vi "Default Settings.vi"(8 "error in (no error)":errorcluster, 11 "8 Inch CAD Dispense in":refnum<class "8 Inch CAD Dispense.lvclass">) -> (0 "error out":errorcluster, 3 "8 Inch CAD Dispense out":refnum<class "8 Inch CAD Dispense.lvclass">)   [LabVIEW 2016, in "8 Inch CAD Dispense.lvclass"]
uses:
  8 Inch CAD Dispense.lvclass
  D:/LabVIEW/20220413/UCSB-Gantry/V5/Classes/Routine/Dispense/CAD Dispense/CAD Dispense.lvclass
  D:/LabVIEW/20220413/UCSB-Gantry/V5/Classes/Routine/Dispense/Dispense.lvclass
  CAD Dispense.lvclass/CAD Dispense.ctl
  Read Glue Speed.vi
  Read Move Speed.vi
  CAD Dispense.lvclass
  Dispense.lvclass
panel:
  # "This Routine does not Accept Settings"
  # "This Routine Does not Accept Settings"
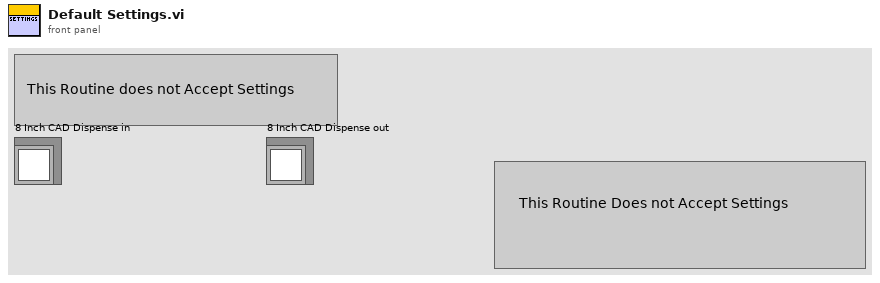
[diagram p1: front panel]
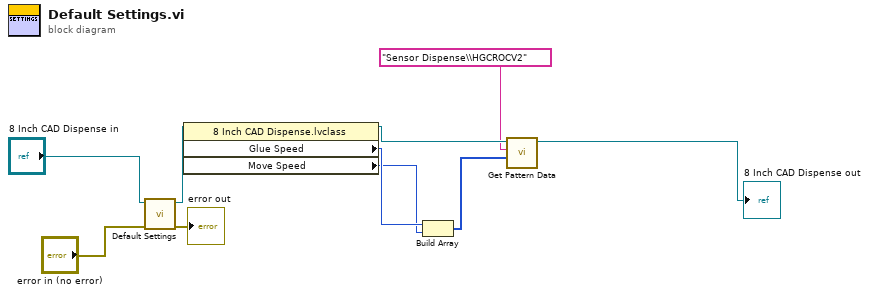
[diagram p0: block diagram]
diagram:
  n1 = call-parent "Default Settings.vi"("error in (no error)"="error in (no error)", "CAD Dispense in"="8 Inch CAD Dispense in") -> ("error out"=→"error out":errorcluster, "CAD Dispense out"=w7:refnum<class "8 Inch CAD Dispense.lvclass">)  [unwired: 8 in]
  n2 = property class="8 Inch CAD Dispense.lvclass"(reference=w7) -> (reference out=w3:refnum<class "8 Inch CAD Dispense.lvclass">, "Glue Speed"=w6:i32, "Move Speed"=w5:i32)  [unwired: 1 in, 1 out]
  n3 = Build Array(w6, w5) -> (w4:i32[])
  n4 = call "Get Pattern Data.vi"("File Name"=w4, "Folder Name"="Sensor Dispense\\HGCROCV2", "Dispense.lvclass"=w3) -> ("Dispense Out"=→"8 Inch CAD Dispense out":refnum<class "8 Inch CAD Dispense.lvclass">)  [unwired: 8 in]
